vi "PostProcessing_LIN_speichern.vi"(8 "error in (no error)":errorcluster caption="Fehler (Eingang, kein Fehler)", 10 "Index active SPAN":i32, 11 "reprocessing index for filname":i32) -> (0 "Fehler (Ausgang)":errorcluster)   [LabVIEW 2020, in "Linearisierung v2.lvlib"]
uses:
  Linearisierung v2.lvlib
  Aktion FGV Post Processing.ctl
  Protokoll/Protokoll.lvlib
  SpanEinstellungen.lvlib
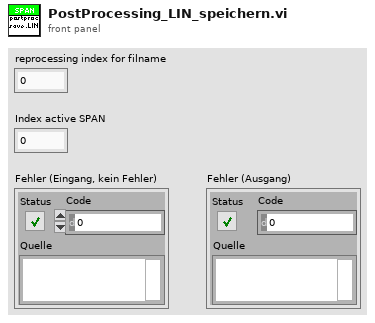
[diagram p1: front panel]
types:
  T1 = typedef "Linearisierung v2.lvlib/Protokoll.lvlib/Aktion LIN Polynom Ordnung ode Aktiv Changes für Postprocessing.ctl" = enum16{"lesen", "schreiben", "init", "init initial"}
  T2 = typedef "Linearisierung v2.lvlib/SpanEinstellungen.lvlib/Aktion FGV Post Processing.ctl" = enum16{"lesen", "set ref", "init", "reset", "enable", "disable", "filenames", "active", "comp", "filename index", "next", "first", "abort", "show"}
  T3 = cluster{"active reprocessing index out":i32, ".LIN Datei Pfad":path}
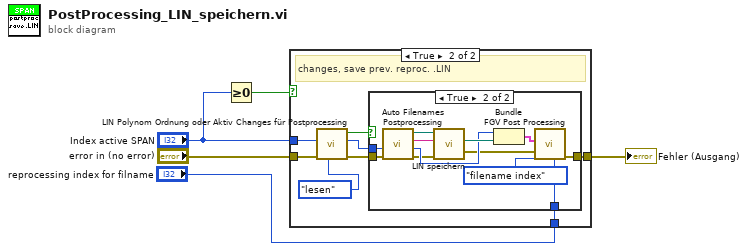
[diagram p0: block diagram]
diagram:
  n1 = Greater Or Equal To 0?(x="Index active SPAN") -> (x >= 0?=w2:bool)
  n2 = case shown="True" w2 {
    tunnel: "Index active SPAN" -> [_ w11]
    tunnel: [w6 w10] -> w5
    tunnel: "error in (no error)" -> [w6 w9]
    tunnel: "reprocessing index for filname" -> [_ w7]
    frame False {
    }
    frame True {
      # "changes, save prev. reproc. .LIN"
      n3 = call "LIN Polynom Ordnung oder Aktiv Changes für Postprocessing.vi"("Aktion"=Aktion_LIN_Polynom_Ordnung_ode_Aktiv_Changes_für_Postprocessing."lesen", "error in (no error)"=w9, "active SPAN Idx"=w11) -> ("error out"=w8:errorcluster, "active SPAN Idx out"=w13:i32, "Changes out"=w14:bool)  [unwired: 5 in, 1 out]
      n4 = case shown="True" w14 {
        tunnel: w13 -> [_ w24]
        tunnel: [w15 w20] -> w10
        tunnel: w8 -> [w15 w19]
        tunnel: w7 -> [_ w16]
        frame False {
        }
        frame True {
          n5 = call "Auto Filenames Postprocessing.vi"("Fehler (Eingang)"=w19, "active postprocessing index"=w24) -> ("Fehler (Ausgang)"=w18:errorcluster, "active reprocessing index out"=w23:i32, "postprocess LIN Filename"=w21:string, "postprocess LIN Pfad"=w22:path)  [unwired: 6 in]
          n6 = call "LIN speichern.vi"("error in (no error)"=w18, "File Name LIN"=w21, "Pfad LIN"=w22) -> ("error out"=w17:errorcluster, ".LIN Datei Pfad"=w26:path)  [unwired: 6 in, 1 out]
          n7 = Bundle("active reprocessing index out"=w23, ".LIN Datei Pfad"=w26) -> (w25:T3)  [unwired: 1 in]
          n8 = call "FGV Post Processing.vi"("reprocessing index for filname"=w16, "Aktion"=Aktion_FGV_Post_Processing."filename index", "error in (no error)"=w17, "filenemas Cluster"=w25) -> ("error out"=w20:errorcluster)  [unwired: 4 in, 3 out]
        }
      }
    }
  }
  "Fehler (Ausgang)" <- w5
